vi "음료자판기(수정).vi"() -> ()   [LabVIEW 2014]
panel:
  in  "음료수량 초기값":cluster{"콜라":u8, "사이다":u8, "생수":u8}={"콜라"=10, "사이다"=10, "생수"=10}
  in  "정지":bool
  in  "구매":bool
  in  "음료":u8(knob) max=2 step=1 scale=0.0..2.0
  out "생수":u8
  out "사이다":u8
  out "콜라":u8
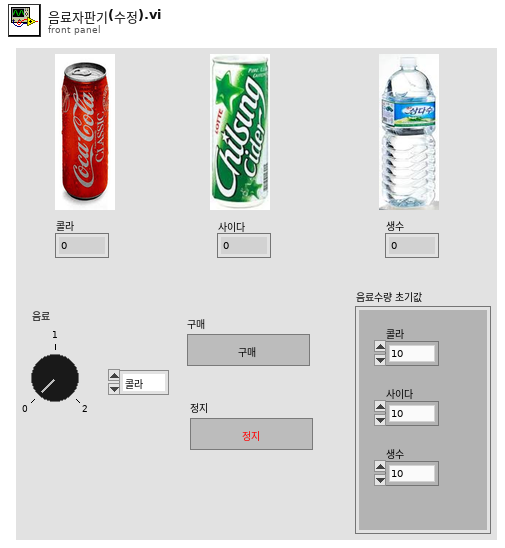
[diagram p1: front panel]
types:
  T1 = typedef "음료.ctl" = enum16{"초기화", "Idle", "구매", "음료확인", "정지"}
  T2 = enum8{"Enabled", "Disabled", "Disabled and Grayed Out"}
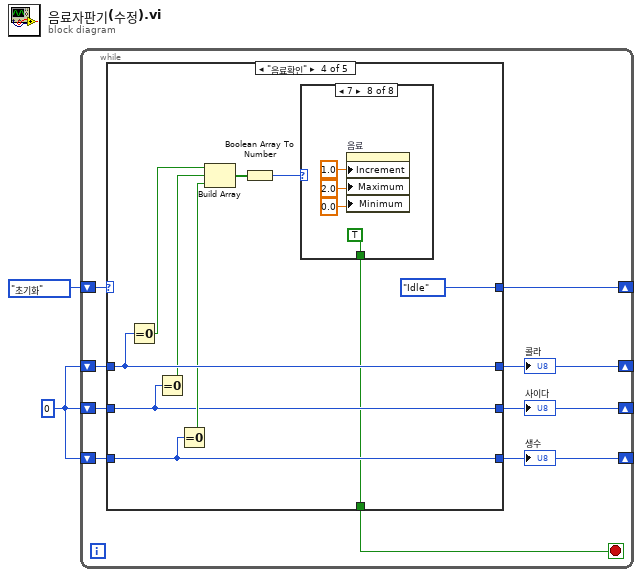
[diagram p0: block diagram]
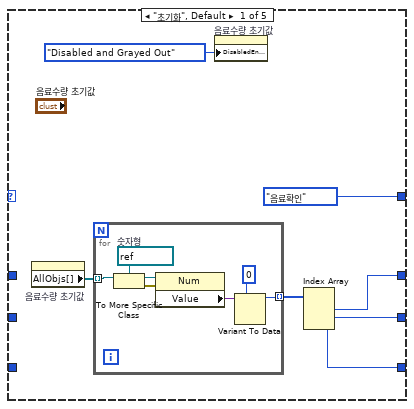
[diagram p2: hidden frame]
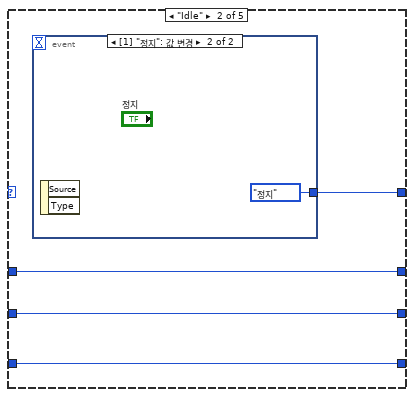
[diagram p3: hidden frame]
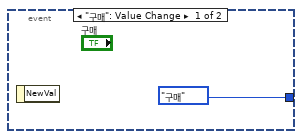
[diagram p4: hidden frame]
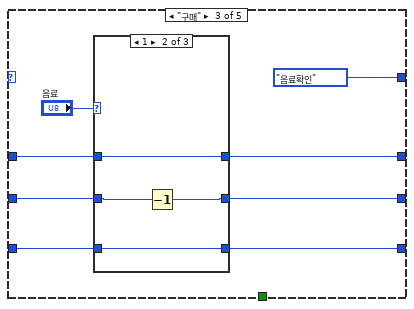
[diagram p5: hidden frame]
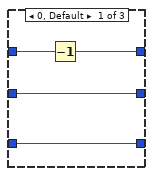
[diagram p6: hidden frame]
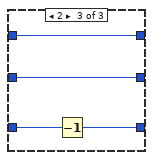
[diagram p7: hidden frame]
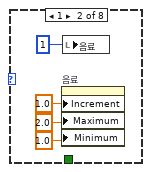
[diagram p9: hidden frame]
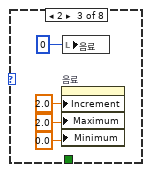
[diagram p10: hidden frame]
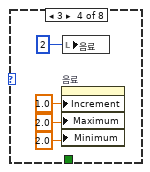
[diagram p11: hidden frame]
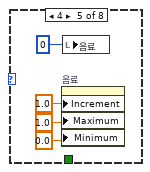
[diagram p12: hidden frame]
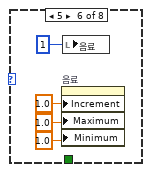
[diagram p13: hidden frame]
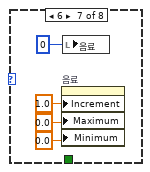
[diagram p14: hidden frame]
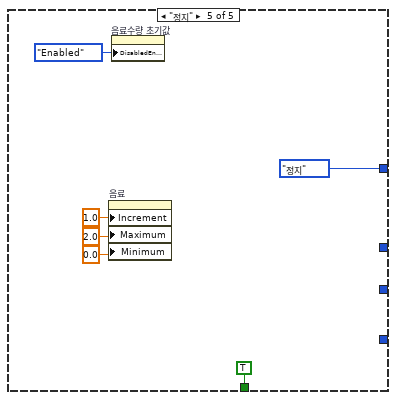
[diagram p15: hidden frame]
diagram:
  w1 = u8 0 ("콜라")
  n1 = while {
    shift-right: [w10] -> _
    shift-left: 음료."초기화" ("열거형") -> [w11]
    shift-right: [w7] -> _
    shift-left: w1 -> [w6]
    shift-right: [w8] -> _
    shift-left: w1 -> [w5]
    shift-right: [w9] -> _
    shift-left: w1 -> [w4]
    stop <- w3 stop-if-true
    n2 = case shown="\"음료확인\"" w11 {
      tunnel: [w14 w29 w36 w60 _] -> w7
      tunnel: [w13 w28 w34 w55 _] -> w8
      tunnel: [w12 w27 w32 w54 _] -> w9
      tunnel: [음료."음료확인" ("열거형") w26 음료."음료확인" ("열거형") 음료."Idle" ("열거형") 음료."정지" ("열거형")] -> w10
      tunnel: w6 -> [_ w29 w37 w60 _]
      tunnel: w5 -> [_ w28 w35 w55 _]
      tunnel: w4 -> [_ w27 w33 w54 _]
      tunnel: [_ _ _ w52 TRUE] -> w3
      frame "초기화", Default {
        n3 = property on="음료수량 초기값" class="Clust (엄격한)"() -> ("AllObjs[]"=w16:refnum<vi>[])  [unwired: 2 in, 2 out]
        n4 = for {
          tunnel: w16 -> [w25] mode=indexing
          tunnel: [w19] -> w15 mode=indexing
          w24 = refnum<vi> refnum  # 숫자형
          n5 = To More Specific Class(target class=w24, reference=w25) -> (specific class reference=w23:refnum<vi>, error out=w22:errorcluster)  [unwired: 1 in]
          n6 = property class="Num"(reference=w23, error in=w22) -> ("Value"=w21:variant)  [unwired: 2 out]
          n7 = Variant To Data(type=u8 0 ("콜라"), Variant=w21) -> (data=w19:u8)  [unwired: 1 in, 1 out]
        }
        n8 = property on="음료수량 초기값" class="Clust (엄격한)"("DisabledEnum"=T2."Disabled and Grayed Out" ("비활성화")) -> ()  [unwired: 2 in, 2 out]
        n9 = Index Array(array=w15) -> (element #1=w14:u8, element #2=w13:u8, element #3=w12:u8)  [unwired: 3 in]
      }
      frame "Idle" {
        n10 = event shown="[1] \"정지\": 값 변경" {
          selector: _ -> [_ _]
          dyn-events: _ -> [_ _]
          timeout: _ -> [_ _]
          tunnel: [음료."구매" ("열거형") 음료."정지" ("열거형")] -> w26
          event "구매": Value Change {
            n11 = event-data() -> ()  [unwired: 1 in, 1 out]
          }
          event "정지": Value Change {
            n12 = event-data() -> ()  [unwired: 1 in, 2 out]
          }
        }
      }
      frame "구매" {
        n13 = case shown="1" "음료" {
          tunnel: w37 -> [w43 w47 w51]
          tunnel: [w42 w47 w51] -> w36
          tunnel: w35 -> [w41 w46 w50]
          tunnel: [w41 w45 w50] -> w34
          tunnel: w33 -> [w40 w44 w49]
          tunnel: [w40 w44 w48] -> w32
          frame 0, Default {
            n14 = Decrement(x=w43) -> (x-1=w42:u8)
          }
          frame 1 {
            n15 = Decrement(x=w46) -> (x-1=w45:u8)
          }
          frame 2 {
            n16 = Decrement(x=w49) -> (x-1=w48:u8)
          }
        }
      }
      frame "음료확인" {
        n17 = Equal To 0?(x=w60) -> (x = 0?=w59:bool)
        n18 = Equal To 0?(x=w55) -> (x = 0?=w58:bool)
        n19 = Equal To 0?(x=w54) -> (x = 0?=w57:bool)
        n20 = Build Array(w59, w58, w57) -> (w56:bool[])
        n21 = Boolean Array To Number(Boolean array=w56) -> (number=w53:u32)
        n22 = case shown="7" w53 {
          tunnel: [_ _ _ _ _ _ _ TRUE] -> w52
          frame 0, Default {
          }
          frame 1 {
            n23 = property on="음료" class="Knob (엄격한)"("Increment"=1.0 ("데이터 입력 제한:증가"), "Maximum"=2.0 ("데이터 입력 제한:최대"), "Minimum"=1.0 ("데이터 입력 제한:최소")) -> ()  [unwired: 2 in, 2 out]
            n24 = local write "음료"(u8 1) -> ()
          }
          frame 2 {
            n25 = property on="음료" class="Knob (엄격한)"("Increment"=2.0 ("데이터 입력 제한:증가"), "Maximum"=2.0 ("데이터 입력 제한:최대"), "Minimum"=0.0 ("데이터 입력 제한:최소")) -> ()  [unwired: 2 in, 2 out]
            n26 = local write "음료"(u8 0) -> ()
          }
          frame 3 {
            n27 = property on="음료" class="Knob (엄격한)"("Increment"=1.0 ("데이터 입력 제한:증가"), "Maximum"=2.0 ("데이터 입력 제한:최대"), "Minimum"=2.0 ("데이터 입력 제한:최소")) -> ()  [unwired: 2 in, 2 out]
            n28 = local write "음료"(u8 2) -> ()
          }
          frame 4 {
            n29 = property on="음료" class="Knob (엄격한)"("Increment"=1.0 ("데이터 입력 제한:증가"), "Maximum"=1.0 ("데이터 입력 제한:최대"), "Minimum"=0.0 ("데이터 입력 제한:최소")) -> ()  [unwired: 2 in, 2 out]
            n30 = local write "음료"(u8 0) -> ()
          }
          frame 5 {
            n31 = property on="음료" class="Knob (엄격한)"("Increment"=1.0 ("데이터 입력 제한:증가"), "Maximum"=1.0 ("데이터 입력 제한:최대"), "Minimum"=1.0 ("데이터 입력 제한:최소")) -> ()  [unwired: 2 in, 2 out]
            n32 = local write "음료"(u8 1) -> ()
          }
          frame 6 {
            n33 = property on="음료" class="Knob (엄격한)"("Increment"=1.0 ("데이터 입력 제한:증가"), "Maximum"=0.0 ("데이터 입력 제한:최대"), "Minimum"=0.0 ("데이터 입력 제한:최소")) -> ()  [unwired: 2 in, 2 out]
            n34 = local write "음료"(u8 0) -> ()
          }
          frame 7 {
            n35 = property on="음료" class="Knob (엄격한)"("Increment"=1.0 ("데이터 입력 제한:증가"), "Maximum"=2.0 ("데이터 입력 제한:최대"), "Minimum"=0.0 ("데이터 입력 제한:최소")) -> ()  [unwired: 2 in, 2 out]
          }
        }
      }
      frame "정지" {
        n36 = property on="음료" class="Knob (엄격한)"("Increment"=1.0 ("데이터 입력 제한:증가"), "Maximum"=2.0 ("데이터 입력 제한:최대"), "Minimum"=0.0 ("데이터 입력 제한:최소")) -> ()  [unwired: 2 in, 2 out]
        n37 = property on="음료수량 초기값" class="Clust (엄격한)"("DisabledEnum"=T2."Enabled" ("비활성화")) -> ()  [unwired: 2 in, 2 out]
      }
    }
    "생수" <- w9
    "사이다" <- w8
    "콜라" <- w7
  }
